vi "FindInstrument.vi"(6 "search string/char ()":string, 8 "error in (no error)":errorcluster) -> (0 "error out":errorcluster, 1 "Found Interface Names":string[](array[string]), 2 "Found Resource Names":string[](array[string]))   [LabVIEW 2013]
doc: "Query the Instruments in the system.\n\nFinds and connects through VISA.\n\nsearch string:\nSearch string can be used to filter results to a particular type that has search string in it Interface Name. It is optional and blank by default.\n\nOutput Found Resource Names are VISA Resource names and Found Interface Names are the matching Interface names.\n\nNote: Rev 2, with a fix to assure not closing existing open instrument sessions while searching."
uses:
  <vilib>/Instr/_visa.llb/VISA Find Search Mode.ctl
panel:
  # "Newport Find Instruments"
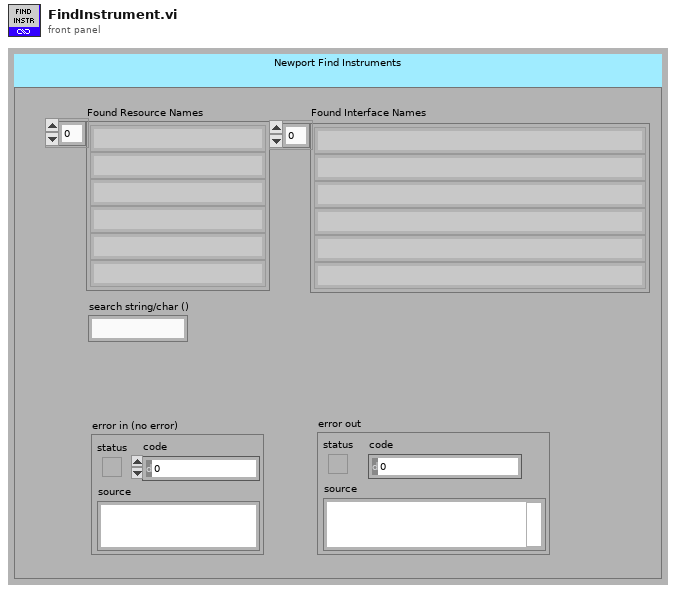
[diagram p1: front panel]
types:
  T1 = typedef "VISA Find Search Mode.ctl" = u32
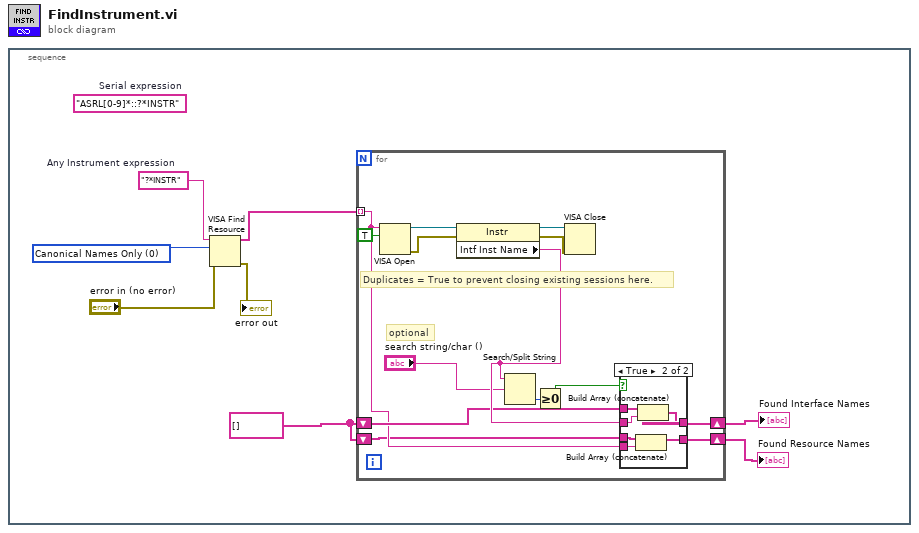
[diagram p0: block diagram]
diagram:
  n1 = stacked-sequence {
    frame #0 {
      (unwired) "ASRL[0-9]*::?*INSTR"  # Serial expression
      w3 = string[] [] ("Array 2")
      w4 = T1 0 items=["Canonical Names Only"=0, "Aliases Only"=2, "Include Matching Aliases"=3, "Include All Aliases"=4] ("Search Mode")
      w5 = "?*INSTR"  # Any Instrument expression
      n2 = VISA Find Resource(8:"error in (no error)", 10:w4, 11:w5) -> (0:→"error out":errorcluster, 3:w7:string[])  [unwired: 1 out]
      n3 = for {
        tunnel: w7 -> [w13] mode=indexing
        shift-right: [w16] -> w6
        shift-left: w3 -> [w14]
        shift-right: [w11] -> w2
        shift-left: w3 -> [w12]
        # "Duplicates = True to prevent closing existing sessions here."
        # "optional"
        n4 = VISA Open(duplicate session (F)=TRUE, VISA resource name=w13) -> (VISA resource name=w22:refnum<visa-resource-name>, error out=w19:errorcluster)  [unwired: 3 in]
        n5 = property class="Instr"(reference=w22, error in=w19) -> (reference out=w21:refnum<visa-resource-name>, error out=w20:errorcluster, "Intf Inst Name"=w15:string)
        n6 = Search/Split String(string=w15, search string/char (-)="search string/char ()") -> (offset of match=w18:i32)  [unwired: 1 in, 2 out]
        n7 = Greater Or Equal To 0?(x=w18) -> (x >= 0?=w17:bool)
        n8 = VISA Close(VISA resource name=w21, error in (no error)=w20) -> ()  [unwired: 1 out]
        n9 = case shown="True" w17 {
          tunnel: w14 -> [w24 w29]
          tunnel: [w24 w30] -> w16
          tunnel: w15 -> [_ w28]
          tunnel: w13 -> [_ w27]
          tunnel: w12 -> [w23 w26]
          tunnel: [w23 w25] -> w11
          frame False {
          }
          frame True {
            n10 = Build Array (concatenate)(w26, w27) -> (w25:string[])
            n11 = Build Array (concatenate)(w29, w28) -> (w30:string[])
          }
        }
      }
      "Found Resource Names" <- w2
      "Found Interface Names" <- w6
    }
  }
